vi "NI_USB6343_DAQmx_DO_PORT_Task_Monitor.vi"(8 "error in (no error)":errorcluster, 11 "VI Server Cluster":T1) -> (0 "error out":errorcluster, 3 "VI Server Cluster.DUP":T1, 5 "task done?":bool)   [LabVIEW 2020]
uses:
  LabVIEW 2020 Toolkits/VI Server Toolkit/VI Server Libraries/VI Server_GetControl.llb/VI Server_DAQmx_PhysicalChannel_Get.vi
  LabVIEW 2020 Toolkits/VI Server Toolkit/VI Server_TypeDefs/VI Server_RefsCluster.ctl
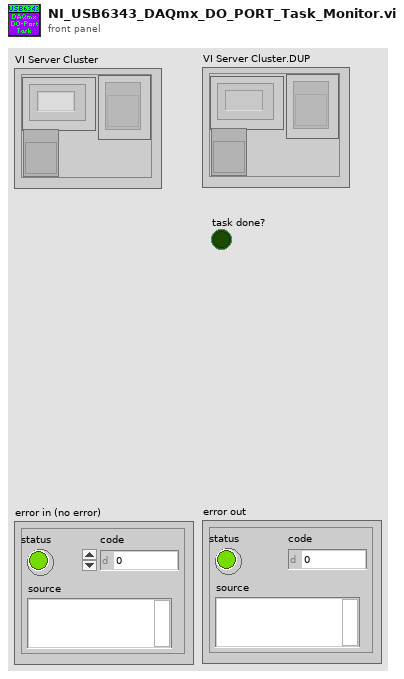
[diagram p1: front panel]
types:
  T1 = typedef "VI Server_RefsCluster.ctl" = cluster{"Labels":string[], "Refs":refnum<vi>[], "VI Ref":refnum<vi>}
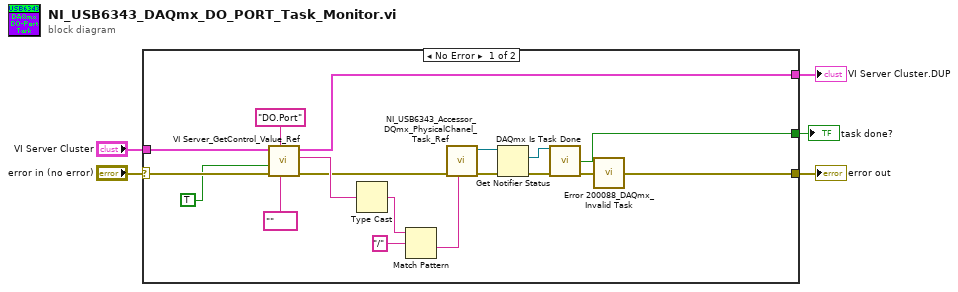
[diagram p0: block diagram]
diagram:
  n1 = case shown="No Error" "error in (no error)" {
    selector: "error in (no error)" -> [w12 w24]
    tunnel: "VI Server Cluster" -> [w13 _]
    tunnel: [w6 w24] -> w4
    tunnel: [w16 _] -> w2
    tunnel: [w8 _] -> w1
    frame No Error {
      n2 = call-poly "VI Server_GetControl_Value_Ref.vi"("DataType"=tag "" ("physical channels"), "Control.Label"="DO.Port", "error in"=w12, "SingleInstance"=TRUE, "VI Server.RefsCluster"=w13) -> ("error out"=w15:errorcluster, "Value"=w22:tag, "VI Server.RefsCluster.DUP"=w16:T1)  [unwired: 3 in, 1 out]
      n3 = Type Cast(x=w22) -> (*(type *) &x=w23:string)  [unwired: 1 in]
      n4 = Match Pattern(string=w23, regular expression="/") -> (after substring=w14:string)  [unwired: 1 in, 3 out]
      n5 = call "NI_USB6343_Accessor_DQmx_PhysicalChanel_Task_Ref.vi"("DAQmx.PhysicalChannel.ID"=w14, "error in (no error)"=w15) -> ("error out"=w18:errorcluster, "DAQmx.TaskNotifier.Ref"=w17:refnum<notifier>)  [unwired: 8 in]
      n6 = Get Notifier Status(notifier=w17, error in (no error)=w18) -> (current notification=w10:refnum<k21>, error out=w9:errorcluster)  [unwired: 3 out]
      n7 = call <vilib>:"DAQmx Is Task Done.vi"("task/channels in"=w10, "error in"=w9) -> ("task done?"=w8:bool, "error out"=w7:errorcluster)  [unwired: 11 in, 1 out]
      n8 = call "Error 200088_DAQmx_Invalid Task.vi"("error in"=w7) -> ("error out"=w6:errorcluster)  [unwired: 13 in, 1 out]
    }
    frame Error {
    }
  }
  "error out" <- w4
  "VI Server Cluster.DUP" <- w2
  "task done?" <- w1
